vi "FTW-JSON-Array-Serialize.vi"(5 "Array of JSON Elements":string[](array[string]), 7 "Whitespace Delimiter (after commas)":string=" ") -> (6 "JSON Array":string)   [LabVIEW 2015]
panel:
  # "Inputs"
  # "Outputs"
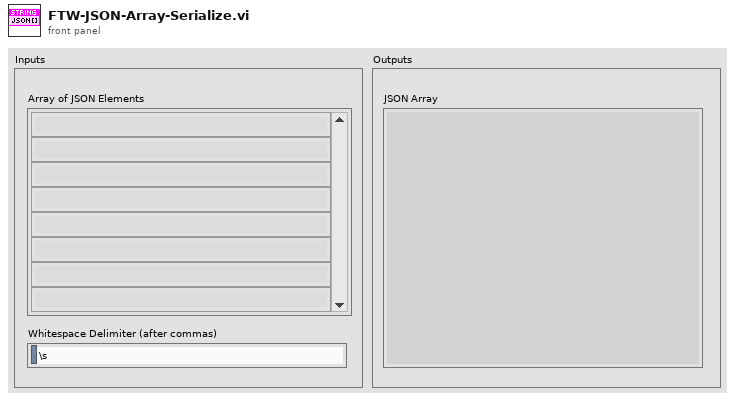
[diagram p1: front panel]
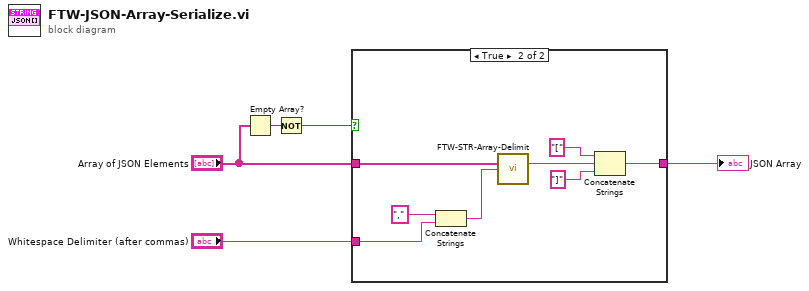
[diagram p0: block diagram]
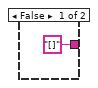
[diagram p2: hidden frame]
diagram:
  n1 = Empty Array?(array="Array of JSON Elements") -> (empty?=w4:bool)
  n2 = Not(x=w4) -> (.not. x?=w3:bool)
  n3 = case shown="True" w3 {
    tunnel: "Array of JSON Elements" -> [_ w14]
    tunnel: "Whitespace Delimiter (after commas)" -> [_ w12]
    tunnel: ["[]" w7] -> w1
    frame False {
    }
    frame True {
      n4 = Concatenate Strings("," ("Delimiter"), w12) -> (w11:string)
      n5 = call "FTW-STR-Array-Delimit.vi"("Array of Strings"=w14, "Delimiter"=w11) -> ("Delimited String"=w10:string)  [unwired: 13 in]
      n6 = Concatenate Strings("[" ("string"), w10, "]" ("string")) -> (w7:string)
    }
  }
  "JSON Array" <- w1
